vi "Enable Heartbeat.vi"(8 "error in":errorcluster, 9 "Period":u32 format="%d ms", 10 "Node ID":u8, 11 "CANopen Actor in":refnum<class "CANopen Actor.lvclass">) -> (0 "error out":errorcluster, 3 "CANopen Actor out":refnum<class "CANopen Actor.lvclass">)   [LabVIEW 2024, in "CANopen Actor.lvlib" / "CANopen Actor.lvclass"]
uses:
  CANopen Actor.lvclass
  CANopen Actor.lvclass/CANopen Actor.ctl
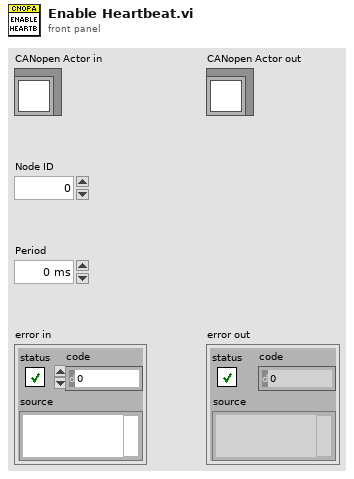
[diagram p1: front panel]
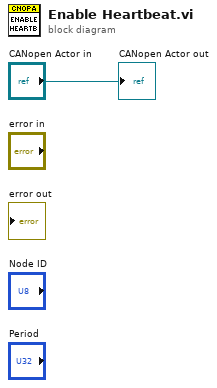
[diagram p0: block diagram]
diagram:
  "CANopen Actor out" <- "CANopen Actor in"
